vi "Stop Sift Proxy.vi"() -> ()   [LabVIEW 2024, in "Sift Client.lvlib"]
doc: "Stop the currently running instance of Sift Proxy. Do not call this unless you need to explicitly stop the process."
uses:
  Sift Client.lvlib
  Sift API/Sift Client.lvclass
panel:
  out "Success":bool
  out "Error":errorcluster
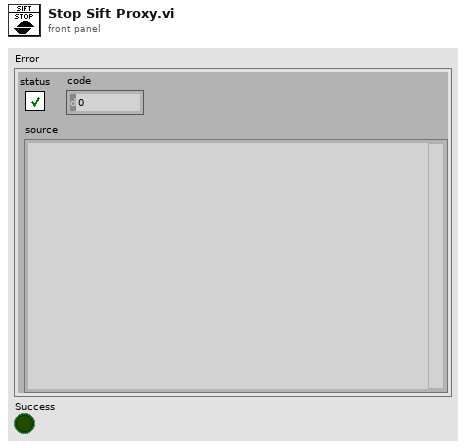
[diagram p1: front panel]
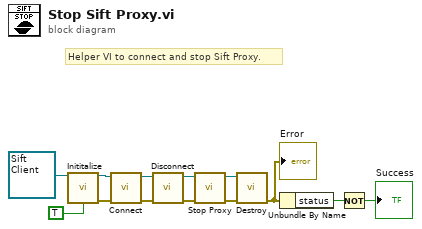
[diagram p0: block diagram]
diagram:
  # "Helper VI to connect and stop Sift Proxy."
  n1 = call-dynamic "Inititalize.vi"("Sift Client in"=refnum<class "Sift Client.lvclass"> refnum ("Sift Client.lvlib:Sift Client.lvclass"), "Test Mode"=TRUE) -> ("Sift Client out"=w10:refnum<class "Sift Client.lvclass">, "error out"=w9:errorcluster)  [unwired: 12 in]
  n2 = call-dynamic "Connect.vi"("error in (no error)"=w9, "Sift Client in"=w10) -> ("error out"=w11:errorcluster, "Sift Client out"=w12:refnum<class "Sift Client.lvclass">)  [unwired: 7 in, 1 out]
  n3 = call-dynamic "Disconnect.vi"("error in (no error)"=w11, "Sift Client in"=w12) -> ("error out"=w6:errorcluster, "Sift Client out"=w8:refnum<class "Sift Client.lvclass">)  [unwired: 8 in]
  n4 = call-dynamic "Stop Proxy.vi"("error in (no error)"=w6, "Sift Client in"=w8) -> ("error out"=w5:errorcluster, "Sift Client out"=w7:refnum<class "Sift Client.lvclass">)  [unwired: 8 in]
  n5 = call-dynamic "Destroy.vi"("error in (no error)"=w5, "Sift Client in"=w7) -> ("error out"=w4:errorcluster)  [unwired: 8 in, 1 out]
  "Error" <- w4
  n6 = Unbundle By Name(w4) -> ("status"=w3:bool)
  n7 = Not(x=w3) -> (.not. x?=→"Success":bool)
